vi "FPGA Write - U8.vi"(8 "error in (no error)":errorcluster, 9 "Value":u8, 10 "Control":T1, 11 "FPGA Session In":refnum<class "Firmware Independent PID Interface.lvclass">) -> (0 "error out":errorcluster, 3 "FPGA Session Out":refnum<class "Firmware Independent PID Interface.lvclass">)   [LabVIEW 2010, in "Firmware Independent PID Interface.lvclass"]
doc: "Writes an unsigned 8-bit integer value to a given control or indicator."
uses:
  Firmware Independent PID Interface.lvclass
  TypeDefs/ControlU8.ctl
  <vilib>/rvi/DataTransferAndStorage/Container/Common/niFpgaDataTypeControl.ctl
  <userlib>/_FPGA Interface Advanced Tools/FPGA Interface Base/FPGA Interface Base.lvclass/FPGA Interface Base.ctl
  <vilib>/Utility/error.llb/Error Cluster From Error Code.vi
  <userlib>/_FPGA Interface Advanced Tools/FPGA Interface Base/Accessors/FPGA Read Session.vi
  <userlib>/_FPGA Interface Advanced Tools/FPGA Interface Wrapper/FPGA Interface Wrapper.lvlib
  <userlib>/_FPGA Interface Advanced Tools/FPGA Interface Base/FPGA Interface Base.lvclass
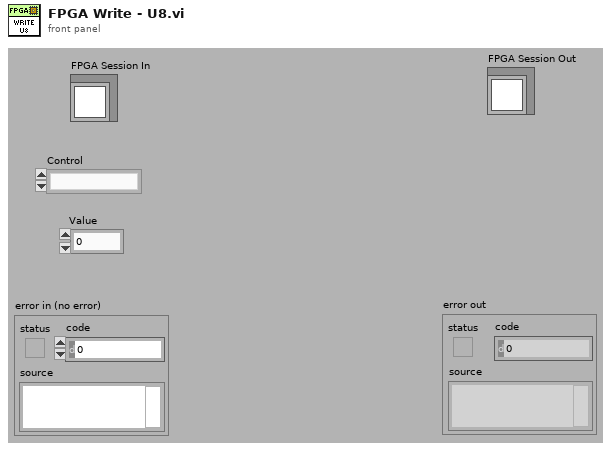
[diagram p1: front panel]
types:
  T1 = typedef "Firmware Independent PID Interface.lvclass/ControlU8.ctl" = enum16{""}
  T2 = typedef "niFpgaDataTypeControl.ctl" = enum32{"Boolean", "I8", "I16", "I32", "I64", "U8", "U16", "U32", "U64", "FXP", "CustomControl"}
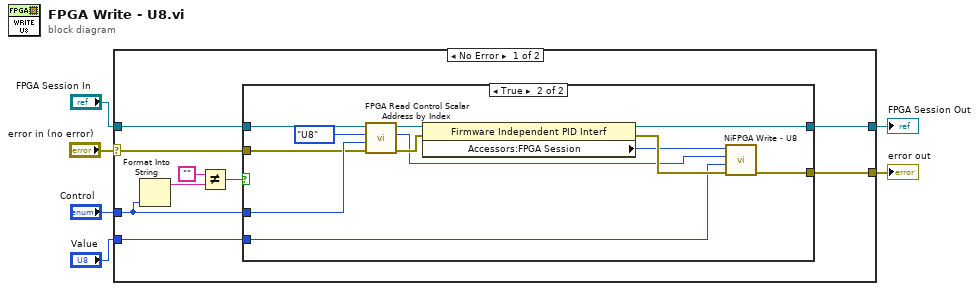
[diagram p0: block diagram]
diagram:
  n1 = case shown="No Error" "error in (no error)" {
    selector: "error in (no error)" -> [w8 w31]
    tunnel: [w10 w31] -> w1
    tunnel: [w9 w30] -> w2
    tunnel: "FPGA Session In" -> [w13 w30]
    tunnel: "Control" -> [w11 _]
    tunnel: "Value" -> [w7 _]
    frame No Error {
      n2 = Format Into String(w11) -> (resulting string=w15:string)  [unwired: 3 in, 1 out]
      n3 = Not Equal?(x="", y=w15) -> (x != y?=w12:bool)
      n4 = case shown="True" w12 {
        tunnel: [w16 w21] -> w10
        tunnel: [w17 w25] -> w9
        tunnel: w13 -> [w17 w26]
        tunnel: w11 -> [_ w24]
        tunnel: w8 -> [w16 w23]
        tunnel: w7 -> [_ w20]
        frame False {
        }
        frame True {
          n5 = call <userlib>:"FPGA Read Control Scalar Address by Index.vi"("error in (no error)"=w23, "index"=w24, "Data Type"=niFpgaDataTypeControl."U8", "FPGA Interface Base in"=w26) -> ("error out"=w28:errorcluster, "Address"=w19:u32, "FPGA Interface Base out"=w27:refnum<class "Firmware Independent PID Interface.lvclass">)  [unwired: 4 in, 1 out]
          n6 = property class="Firmware Independent PID Interf"(reference=w27, error in=w28) -> (reference out=w25:refnum<class "Firmware Independent PID Interface.lvclass">, error out=w22:errorcluster, "Accessors:FPGA Session"=w18:u32)
          n7 = call <userlib>:"NiFPGA Write - U8.vi"("error in (no error)"=w22, "Value"=w20, "Control"=w19, "Session"=w18) -> ("error out"=w21:errorcluster)  [unwired: 6 in, 1 out]
        }
      }
    }
    frame Error {
    }
  }
  "error out" <- w1
  "FPGA Session Out" <- w2
